vi "Dequeue all TDCHits.vi"(8 "error in (no error)":errorcluster, 11 "Queue in":refnum<queue>) -> (0 "error out":errorcluster, 1 "elements dequeued":i32, 2 "TDCHits":T1[](array[typedef]), 3 "Queue out":refnum<queue>)   [LabVIEW 2016]
uses:
  HPTDC Driver Library Folder/Library files/Typedefs/TDCHit.ctl
  HPTDC Driver Library Folder/HPTDC Driver Library.lvlib
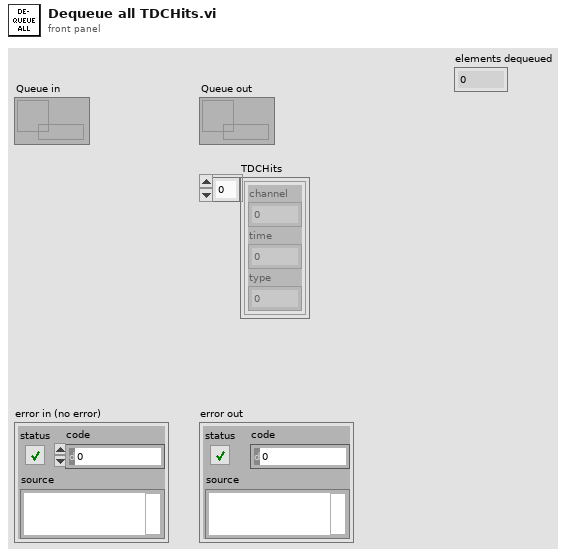
[diagram p1: front panel]
types:
  T1 = typedef "HPTDC Driver Library.lvlib/TDCHit.ctl" = cluster{"channel":u8, "time":u64, "type":u8}
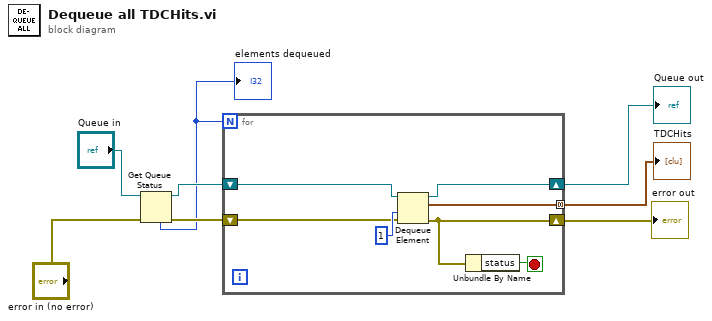
[diagram p0: block diagram]
diagram:
  n1 = Get Queue Status(queue="Queue in", error in (no error)="error in (no error)") -> (queue out=w3:refnum<queue>, error out=w4:errorcluster, # elements in queue=w1:i32)  [unwired: 1 in, 5 out]
  "elements dequeued" <- w1
  n2 = for {
    N: w1 -> [_]
    shift-right: [w14] -> w7
    shift-left: w4 -> [w12]
    tunnel: [w9] -> w2 mode=concatenating
    shift-right: [w15] -> w8
    shift-left: w3 -> [w11]
    stop <- w10 stop-if-true
    n3 = Dequeue Element(queue=w11, timeout in ms (-1)=1, error in (no error)=w12) -> (queue out=w15:refnum<queue>, element=w9:T1[], error out=w14:errorcluster)  [unwired: 1 out]
    n4 = Unbundle By Name(w14) -> ("status"=w10:bool)
  }
  "Queue out" <- w8
  "error out" <- w7
  "TDCHits" <- w2
